vi "Download.vi"(5 "ICAN":refnum<class "ICAN.lvclass">, 7 "Node-ID":u8, 8 "error in":errorcluster, 9 "Value":variant, 10 "Multiplexer":cluster{"Index":u16, "Sub-Index":u8} {"Index" format="%.0x"}, 11 "SDO Manager in":refnum<class "SDO Manager.lvclass">) -> (0 "error out":errorcluster, 2 "Success?":bool, 3 "SDO Manager out":refnum<class "SDO Manager.lvclass">)   [LabVIEW 2024, in "CANopen Master.lvlib" / "SDO Manager.lvclass"]
uses:
  SDO Manager.lvclass
  HAL/HAL/Protocols/ICAN/ICAN.lvclass
  CANopen Message/CANopen Message.lvclass/CANopen Message.ctl
  SDO Manager.lvclass/SDO Manager.ctl
  Service Data Object/Service Data Object.lvclass
  CANopen Message/CANopen Message.lvclass
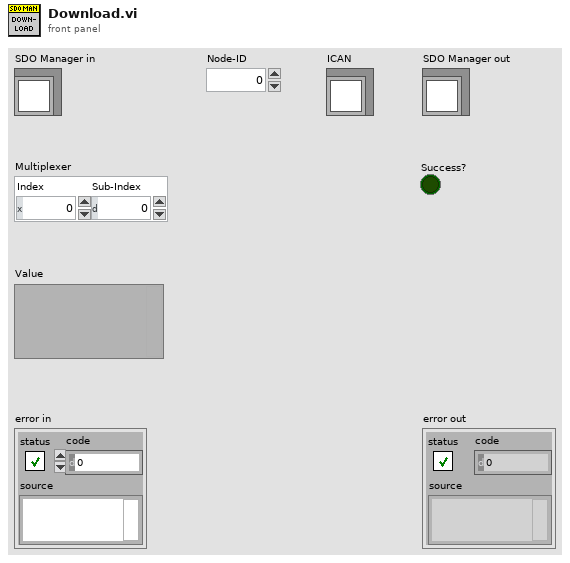
[diagram p1: front panel]
types:
  T1 = typedef "CANopen Master.lvlib/SDO Manager.lvclass/ObjectAttributes.ctl" = cluster{"SDO Response Map":map{u32, refnum<notifier>}}
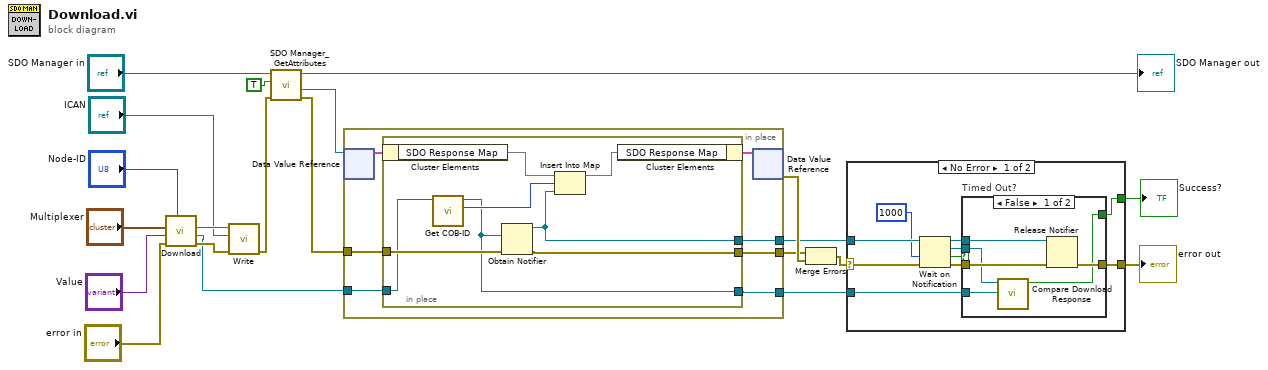
[diagram p0: block diagram]
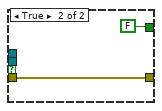
[diagram p2: hidden frame]
diagram:
  n1 = call "Download.vi"("Node-ID"="Node-ID", "error in"="error in", "Value"="Value", "Multiplexer"="Multiplexer") -> ("error out"=w9:errorcluster, "CANopen Response Message"=w8:refnum<class "CANopen Message.lvclass">, "CANopen Message"=w11:refnum<class "CANopen Message.lvclass">)  [unwired: 4 in, 1 out]
  n2 = call "Write.vi"("error in"=w9, "ICAN"="ICAN", "CANopen Message in"=w11) -> ("error out"=w3:errorcluster)  [unwired: 7 in, 1 out]
  n3 = call "SDO Manager_GetAttributes.vi"("Error In"=w3, "OnlyGetDvrReference(False)"=TRUE, "reference in"="SDO Manager in") -> ("Error Out"=w2:errorcluster, "DataRef"=w17:refnum<data-value>, "reference out"=→"SDO Manager out":refnum<class "SDO Manager.lvclass">)  [unwired: 5 in, 1 out]
  n4 = in-place {
    in-place-border: [w28] -> w14
    in-place-border: w2 -> [w27]
    in-place-border: w8 -> [w26]
    in-place-border: [w22] -> w7
    in-place-border: [w25] -> w5
    n5 = in-place-dvr #1(w17) -> (w24:T1)  [unwired: 1 out]
    n6 = in-place {
      in-place-border: [w36] -> w28
      in-place-border: w27 -> [w34]
      in-place-border: w26 -> [w30]
      in-place-border: [w33] -> w25
      in-place-border: [w29] -> w22
      n7 = in-place-cluster #2(w24) -> ("SDO Response Map"=w32:map{u32, refnum<notifier>})
      n8 = call "Get COB-ID.vi"("CANopen Message in"=w30) -> ("COB-ID"=w35:u32, "CANopen Message out"=w29:refnum<class "CANopen Message.lvclass">)  [unwired: 9 in]
      n9 = Obtain Notifier(notification data type=w29, error in (no error)=w34) -> (notifier out=w36:refnum<notifier>, error out=w33:errorcluster)  [unwired: 2 in, 1 out]
      n10 = Insert Into Map(map in=w32, key=w35, value=w36) -> (map out=w31:map{u32, refnum<notifier>})  [unwired: 2 out]
      n11 = in-place-cluster #2("SDO Response Map"=w31) -> (w23:T1)
    }
    n12 = in-place-dvr #1(w23) -> (w15:errorcluster)  [unwired: 1 out]
  }
  n13 = Merge Errors(w5, w15) -> (w6:errorcluster)
  n14 = case shown="No Error" w6 {
    selector: w6 -> [w44 w55]
    tunnel: w14 -> [w46 _]
    tunnel: [w41 w55] -> w13
    tunnel: [w38 _] -> w12
    tunnel: w7 -> [w39 _]
    frame No Error {
      n15 = Wait on Notification(notifier=w46, timeout in ms (-1)=1000, error in (no error)=w44) -> (notifier out=w43:refnum<notifier>, notification=w40:refnum<class "CANopen Message.lvclass">, timed out?=w37:bool, error out=w42:errorcluster)  [unwired: 1 in]
      n16 = case "Timed Out?" shown="False" w37 {
        tunnel: w43 -> [w52 _]
        tunnel: w42 -> [w51 w54]
        tunnel: [w50 w54] -> w41
        tunnel: w40 -> [w49 _]
        tunnel: w39 -> [w48 _]
        tunnel: [w47 FALSE ("Equal?")] -> w38
        frame False {
          n17 = call "Compare Download Response.vi"("Expected"=w48, "Actual"=w49) -> ("Equal?"=w47:bool)  [unwired: 9 in]
          n18 = Release Notifier(notifier=w52, error in (no error)=w51) -> (error out=w50:errorcluster)  [unwired: 1 in, 2 out]
        }
        frame True {
        }
      }
    }
    frame Error {
    }
  }
  "error out" <- w13
  "Success?" <- w12
